vi "Handle Processing Error.vi"(8 "error in (no error)":errorcluster, 11 "StreamReader in":refnum<class "StreamReader.lvclass">) -> (0 "error out":errorcluster, 2 "Error Response":T1, 3 "StreamReader out":refnum<class "StreamReader.lvclass">)   [LabVIEW 2024, in "StreamReader.lvlib" / "StreamReader.lvclass"]
uses:
  StreamReader.lvclass
  StreamReader.lvclass/StreamReader.ctl
  <vilib>/FlexLogger/SDK/PluginSDK.lvlibp/PEFClasses/SDK/Processing Element/Error Response Type.ctl
  <vilib>/FlexLogger/SDK/PluginSDK.lvlibp/PEFClasses/SDK/Processing Element/Processing Element.lvclass
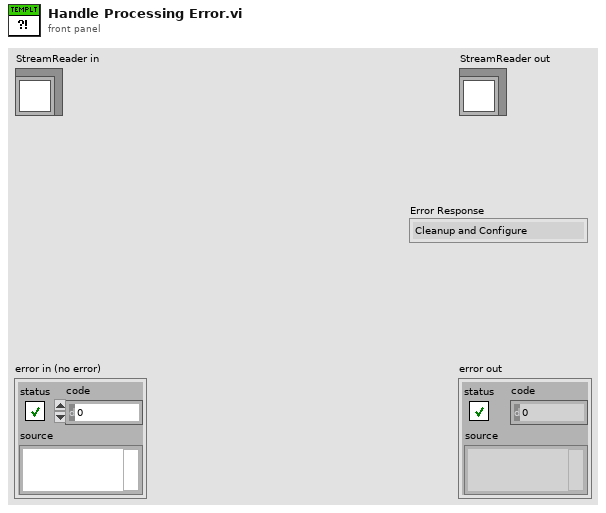
[diagram p1: front panel]
types:
  T1 = typedef "PluginSDK.lvlibp/Processing Element.lvclass/Error Response Type.ctl" = enum16{"Cleanup and Configure", "Cleanup and Finalize", "Report and Continue"}
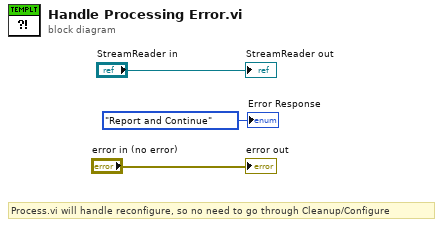
[diagram p0: block diagram]
diagram:
  # "Process.vi will handle reconfigure, so no need to go through Cleanup/Configure"
  "error out" <- "error in (no error)"
  "StreamReader out" <- "StreamReader in"
  "Error Response" <- Error_Response_Type."Report and Continue" ("Error Response")
